vi "Volume_Naming.vi"() -> (5 "Plug in titles":string[](array[string]), 7 "Plug in values":string[](array[string]))   [LabVIEW 2013]
uses:
  File/Setup_Filetype.ctl
  Globals/Meas_global.vi
panel:
  out "Volume File Present?":bool=TRUE
  out "Values":string[](array[string])
  out "Output Position":dbl[](array[numeric])
  out "Zmin":dbl
  out "Ymin":dbl
  out "Zmax":dbl
  out "Ymax":dbl
  out "Z":dbl
  out "Volume Name":string
  out "Y":dbl
  out "X":dbl
  out "Row number":i32
  out "Xmin":dbl
  out "Xmax":dbl
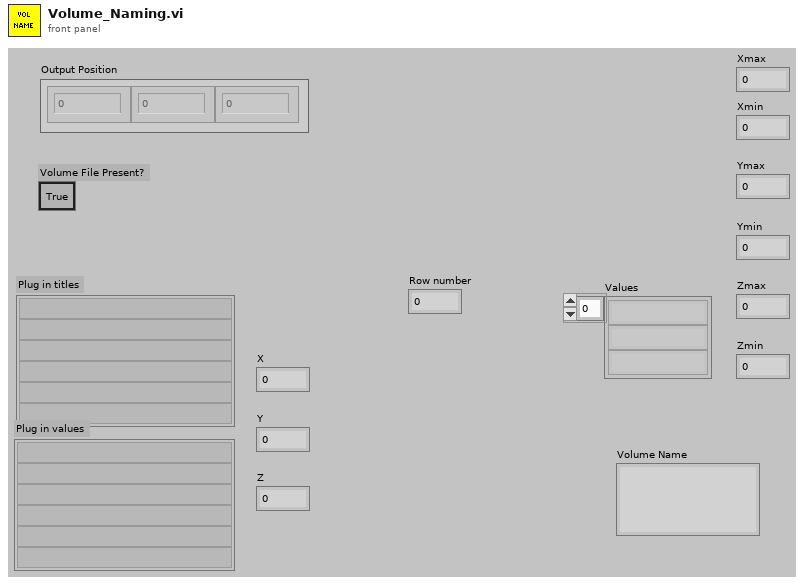
[diagram p1: front panel]
types:
  T1 = typedef "Setup_Filetype.ctl" = enum16{"Measurement Setups", "Calibration Setups", "General", "Results File Plotter Setups", "Speed Calib Tweaks"}
  T2 = enum16{"To Traverse Coordinates", "To User Coordinates"}
  T3 = typedef "Post_Process.ctl" = enum16{"Take New Data", "Post Process Raw Data File"}
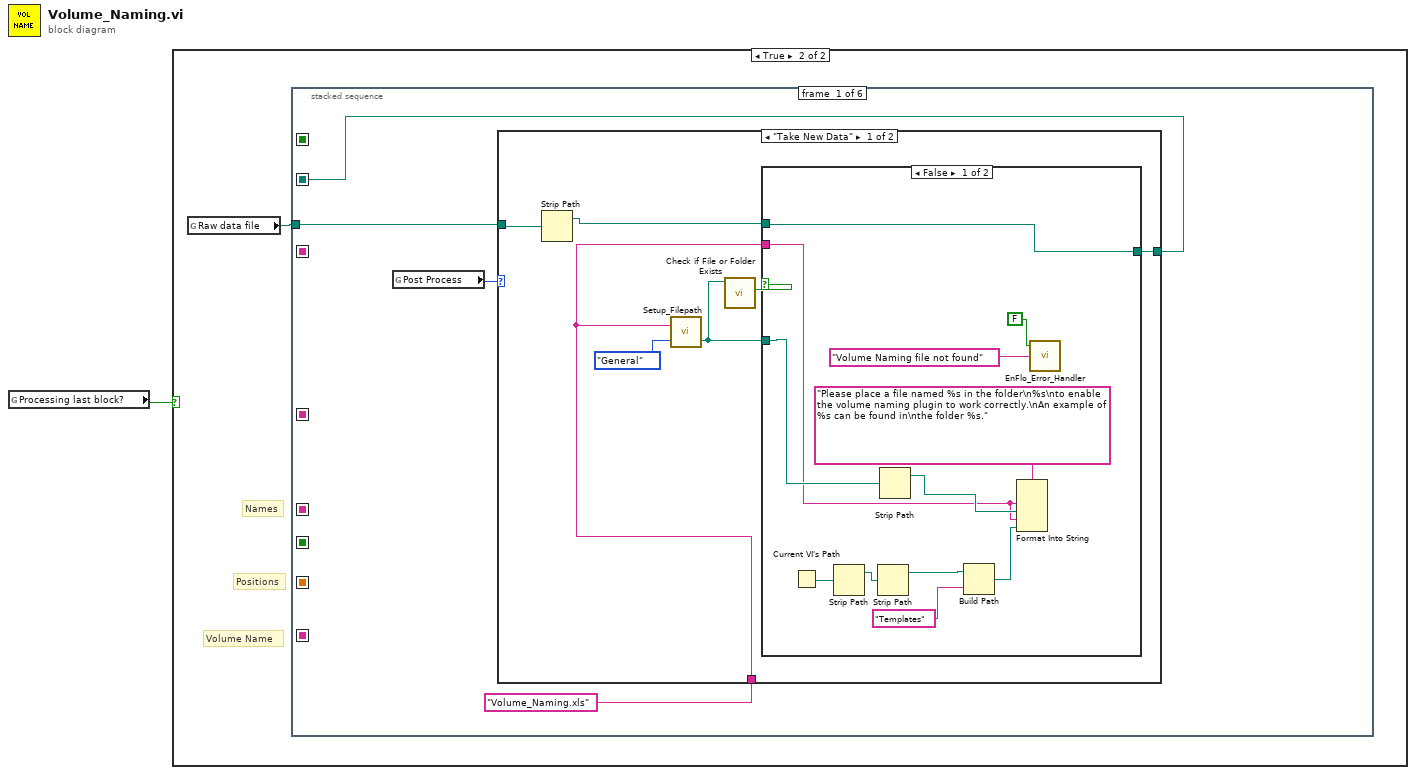
[diagram p0: block diagram]
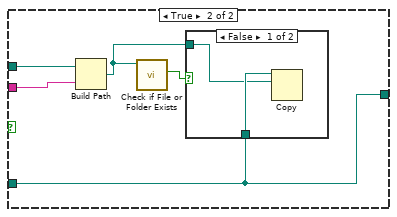
[diagram p3: hidden frame]
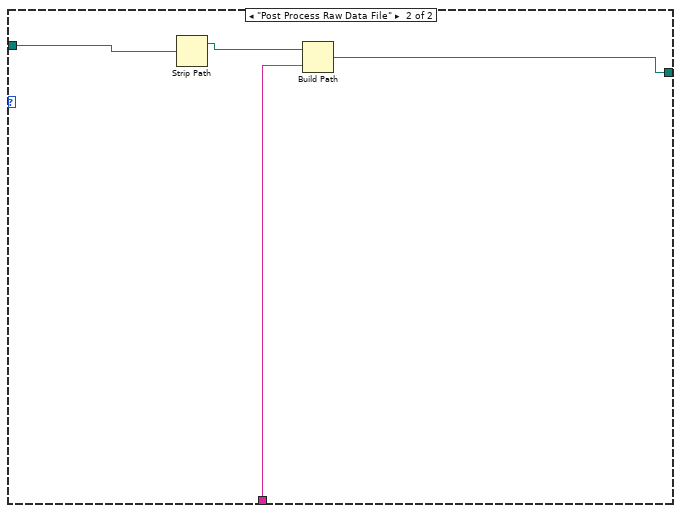
[diagram p5: hidden frame]
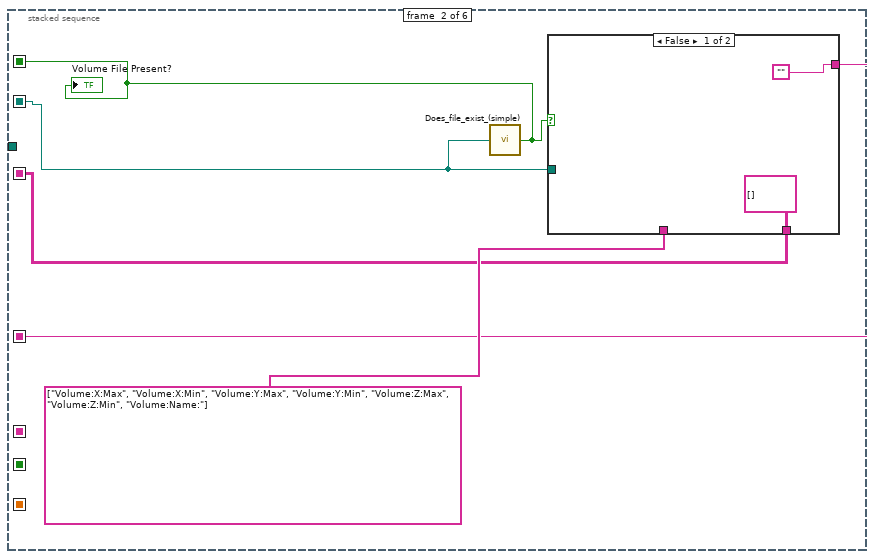
[diagram p6: hidden frame]
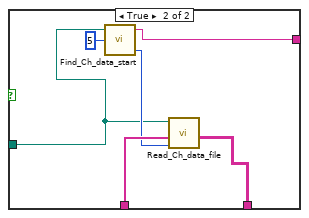
[diagram p7: hidden frame]
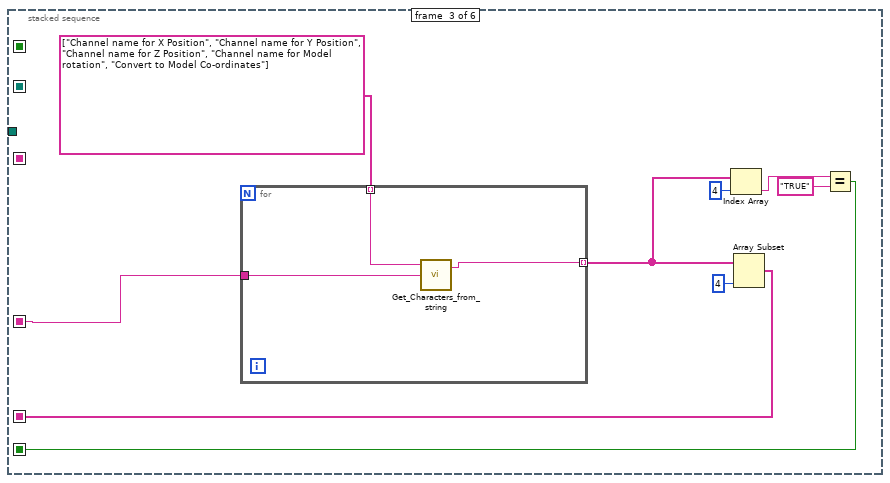
[diagram p8: hidden frame]
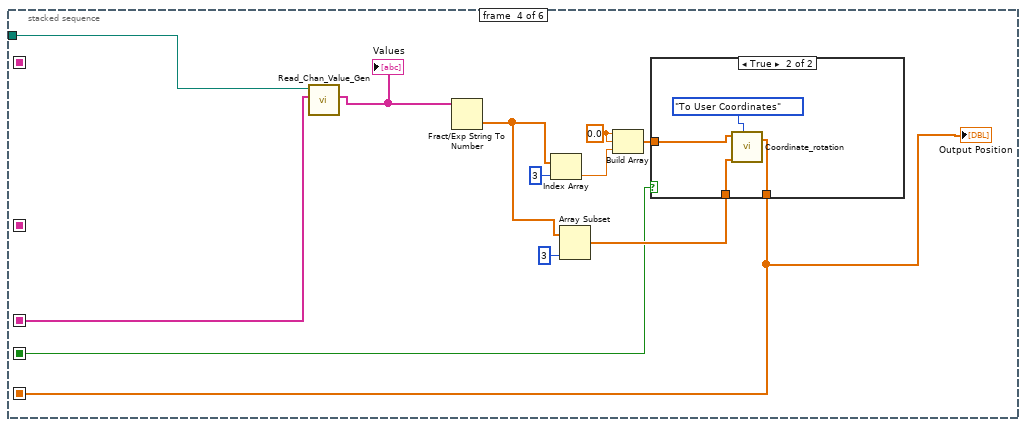
[diagram p9: hidden frame]
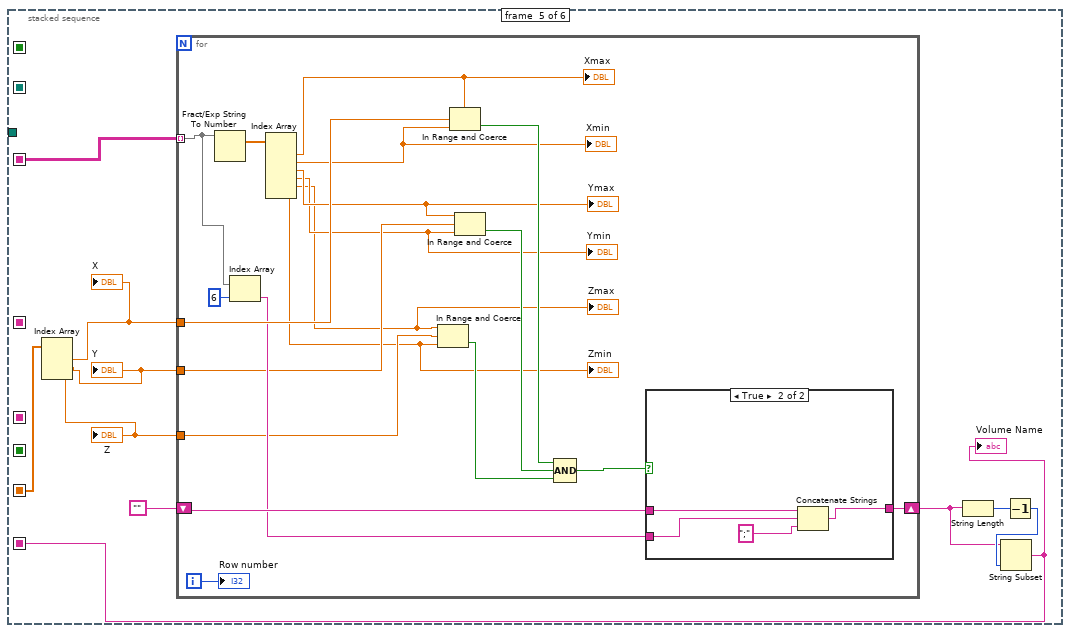
[diagram p11: hidden frame]
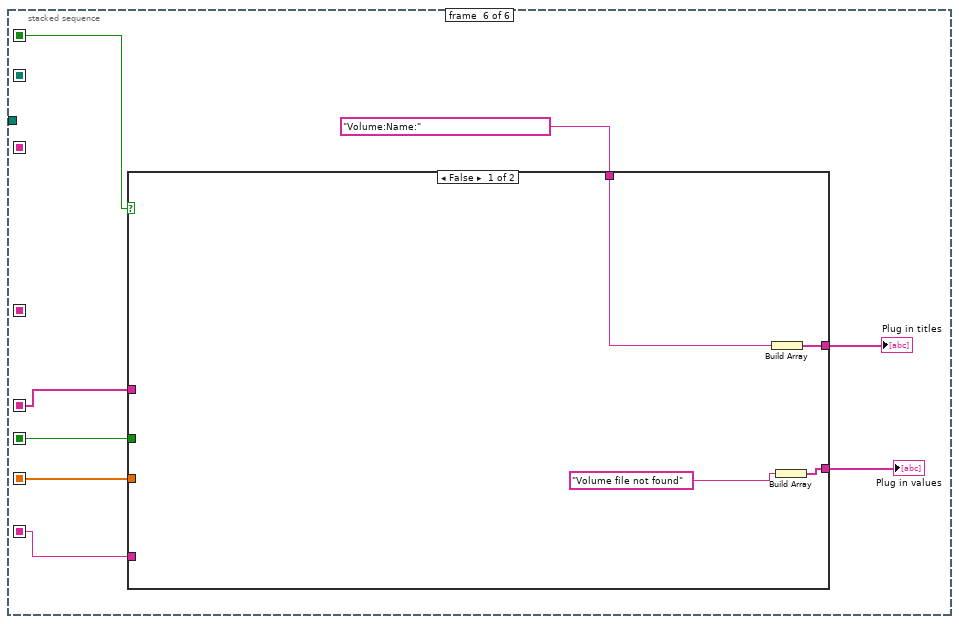
[diagram p13: hidden frame]
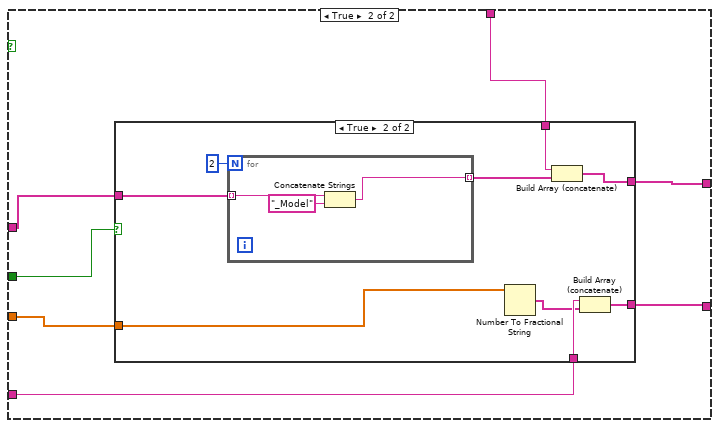
[diagram p14: hidden frame]
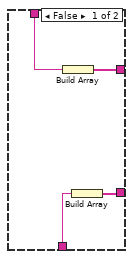
[diagram p15: hidden frame]
diagram:
  n1 = global read "Meas_global.vi" "Processing last block?"() -> (w1:bool)
  n2 = case shown="True" w1 {
    frame False {
    }
    frame True {
      # "Volume Name"
      # "Positions"
      # "Names"
      n3 = global read "Meas_global.vi" "Raw data file"() -> (w2:path)
      n4 = stacked-sequence {
        seq-local: [_ w40 _ _ _ _] -> [_ _ _ _ w88 _]
        seq-local: [_ _ _ w63 _ _] -> [_ _ _ _ w86 w121]
        seq-local: [_ _ _ _ w79 _] -> [_ _ _ _ _ w119]
        seq-local: [_ w39 _ _ _ _] -> [_ _ w58 _ _ _]
        seq-local: [_ _ w55 _ _ _] -> [_ _ _ w65 _ w116]
        seq-local: [_ _ w50 _ _ _] -> [_ _ _ w64 _ w120]
        seq-local: [_ w38 _ _ _ _] -> [_ _ _ _ _ w115]
        seq-local: [w5 _ _ _ _ _] -> [_ w37 _ _ _ _]
        tunnel: w2 -> [w4 _ _ w62 _ _]
        frame #0 {
          n5 = global read "Meas_global.vi" "Post Process"() -> (w6:T3)
          n6 = case shown="\"Take New Data\"" w6 {
            tunnel: [w7 w33] -> w5
            tunnel: w4 -> [w12 w35]
            tunnel: "Volume_Naming.xls" ("name or relative path") -> [w10 w34]
            frame "Take New Data" {
              n7 = Strip Path(path=w12) -> (stripped path=w11:path)  [unwired: 1 out]
              n8 = call "Setup_Filepath.vi"("Setup File Type"=Setup_Filetype."General", "Filename in"=w10) -> ("Filename Out"=w9:path)  [unwired: 1 out]
              n9 = call <vilib>:"Check if File or Folder Exists.vi"("path"=w9) -> ("file or folder exists?"=w8:bool)  [unwired: 8 in, 2 out]
              n10 = case shown="False" w8 {
                tunnel: w11 -> [w14 w30]
                tunnel: w10 -> [w20 w29]
                tunnel: w9 -> [w22 w26]
                tunnel: [w14 w26] -> w7
                frame False {
                  n11 = Current VI's Path() -> (path=w19:path)
                  n12 = Strip Path(path=w19) -> (stripped path=w18:path)  [unwired: 1 out]
                  n13 = Strip Path(path=w18) -> (stripped path=w17:path)  [unwired: 1 out]
                  n14 = Strip Path(path=w22) -> (stripped path=w21:path)  [unwired: 1 out]
                  n15 = Build Path(base path=w17, name or relative path="Templates") -> (appended path=w15:path)
                  n16 = Format Into String(format string="Please place a file named %s in the folder\n%s\nto enable the volume naming plugin to work correctly.\nAn example of %s can be found in\nthe folder %s.", w20, w21, w20, w15) -> ()  [unwired: 2 in, 2 out]
                  n17 = call "EnFlo_Error_Handler.vi"("Error Type"="Volume Naming file not found", "Dialog Box (T)"=FALSE) -> ()  [unwired: 1 in, 3 out]
                }
                frame True {
                  n18 = Build Path(base path=w30, name or relative path=w29) -> (appended path=w27:path)
                  n19 = call <vilib>:"Check if File or Folder Exists.vi"("path"=w27) -> ("file or folder exists?"=w28:bool)  [unwired: 8 in, 2 out]
                  n20 = case shown="False" w28 {
                    tunnel: w26 -> [w32 _]
                    tunnel: w27 -> [w31 _]
                    frame False {
                      n21 = Copy(10:w31, 11:w32) -> ()  [unwired: 3 in, 3 out]
                    }
                    frame True {
                    }
                  }
                }
              }
            }
            frame "Post Process Raw Data File" {
              n22 = Strip Path(path=w35) -> (stripped path=w36:path)  [unwired: 1 out]
              n23 = Build Path(base path=w36, name or relative path=w34) -> (appended path=w33:path)
            }
          }
        }
        frame #1 {
          n24 = call "Does_file_exist_(simple).vi"("Pathname"=w37) -> ("exists?"=w38:bool)
          "Volume File Present?" <- w38
          n25 = case shown="False" w38 {
            tunnel: string[] ["Volume:X:Max", "Volume:X:Min", "Volume:Y:Max", "Volume:Y:Min", "Volume:Z:Max", "Volume:Z:Min", "Volume:Name:"] ("Ch names Out") -> [_ w49]
            tunnel: [string[][] [] ("Channel Values") w48] -> w40
            tunnel: ["" w47] -> w39
            tunnel: w37 -> [_ w44]
            frame False {
            }
            frame True {
              n26 = call "Find_Ch_data_start.vi"("Approx No Of Columns"=5, "Filename"=w44) -> ("Start of read offset output"=w45:i32, "String before data"=w47:string)  [unwired: 1 in, 1 out]
              n27 = call "Read_Ch_data_file.vi"("Start of read offset (chars.: 0)"=w45, "Present Channels"=w49, "Filename"=w44) -> ("Channel Values"=w48:string[][])  [unwired: 2 in, 4 out]
            }
          }
        }
        frame #2 {
          n28 = for {
            tunnel: w58 -> [w61]
            tunnel: string[] ["Channel name for X Position", "Channel name for Y Position", "Channel name for Z Position", "Channel name for Model rotation", "Convert to Model Co-ordinates"] -> [w60] mode=indexing
            tunnel: [w59] -> w54 mode=indexing
            n29 = call "Get_Characters_from_string.vi"("Input string"=w61, "Variable name"=w60) -> ("Value"=w59:string)  [unwired: 1 in, 1 out]
          }
          n30 = Index Array(array=w54, index=4) -> (element=w52:string)
          n31 = Array Subset(array=w54, length=4) -> (w55:string[])  [unwired: 1 in]
          n32 = Equal?(x=w52, y="TRUE") -> (x = y?=w50:bool)
        }
        frame #3 {
          w70 = 0.0 ("element")
          n33 = call "Read_Chan_Value_Gen.vi"("Desired Ch Names"=w65, "Raw data file"=w62) -> ("Values"=w73:string[])  [unwired: 9 in]
          "Values" <- w73
          n34 = Fract/Exp String To Number(string=w73) -> (number=w68:dbl[])  [unwired: 3 in, 1 out]
          n35 = Index Array(array=w68, index=3) -> (element=w71:dbl)
          n36 = Array Subset(array=w68, length=3) -> (w66:dbl[])  [unwired: 1 in]
          n37 = Build Array(w70, w70, w71) -> (w69:dbl[])
          n38 = case shown="True" w64 {
            tunnel: w69 -> [_ w77]
            tunnel: w66 -> [w74 w76]
            tunnel: [w74 w75] -> w63
            frame False {
            }
            frame True {
              n39 = call "Coordinate_rotation.vi"("Model       Roll      Pitch       Yaw (deg)"=w77, "Input Position"=w76, "Mode"=T2."To User Coordinates") -> ("Output Position"=w75:dbl[])  [unwired: 2 in, 1 out]
            }
          }
          "Output Position" <- w63
        }
        frame #4 {
          n40 = Index Array(array=w86) -> (element #1=w85:dbl, element #2=w84:dbl, element #3=w83:dbl)  [unwired: 3 in]
          "X" <- w85
          "Y" <- w84
          "Z" <- w83
          n41 = for {
            tunnel: w88 -> [w106] mode=indexing
            tunnel: w85 -> [w103]
            shift-right: [w98] -> w80
            shift-left: "" -> [w100]
            tunnel: w84 -> [w94]
            tunnel: w83 -> [w92]
            i -> [w108]
            n42 = Fract/Exp String To Number(string=w106) -> (number=w107:dbl[])  [unwired: 3 in, 1 out]
            n43 = Index Array(array=w106, index=6) -> (element=w99:string)
            n44 = Index Array(array=w107) -> (element #1=w104:dbl, element #2=w97:dbl, element #3=w95:dbl, element #4=w93:dbl, element #5=w89:dbl, element #6=w90:dbl)  [unwired: 6 in]
            "Xmax" <- w104
            "Xmin" <- w97
            "Ymax" <- w95
            "Zmax" <- w89
            "Ymin" <- w93
            "Zmin" <- w90
            n45 = In Range and Coerce(upper limit=w89, x=w92, lower limit=w90) -> (In Range?=w91:bool)  [unwired: 1 out]
            n46 = In Range and Coerce(upper limit=w104, x=w103, lower limit=w97) -> (In Range?=w102:bool)  [unwired: 1 out]
            n47 = In Range and Coerce(upper limit=w95, x=w94, lower limit=w93) -> (In Range?=w96:bool)  [unwired: 1 out]
            n48 = Compound Arithmetic op=AND(w102, w96, w91) -> (w101:bool)
            n49 = case shown="True" w101 {
              tunnel: w100 -> [w109 w113]
              tunnel: w99 -> [_ w112]
              tunnel: [w109 w110] -> w98
              frame False {
              }
              frame True {
                n50 = Concatenate Strings(w113, w112, ";") -> (w110:string)
              }
            }
            "Row number" <- w108
          }
          n51 = String Length(string=w80) -> (length=w82:i32)
          n52 = Decrement(x=w82) -> (x-1=w81:i32)
          n53 = String Subset(string=w80, length (rest)=w81) -> (substring=w79:string)  [unwired: 1 in]
          "Volume Name" <- w79
        }
        frame #5 {
          n54 = case shown="False" w115 {
            tunnel: w121 -> [_ w132]
            tunnel: w120 -> [_ w131]
            tunnel: w119 -> [_ w130]
            tunnel: [w124 w129] -> w118
            tunnel: [w123 w128] -> w117
            tunnel: w116 -> [_ w127]
            tunnel: "Volume:Name:" -> [w125 w126]
            frame False {
              n55 = Build Array(w125) -> (w124:string[])
              n56 = Build Array("Volume file not found") -> (w123:string[])
            }
            frame True {
              n57 = case shown="True" w131 {
                tunnel: w132 -> [_ w145]
                tunnel: w126 -> [w136 w144]
                tunnel: w130 -> [w133 w143]
                tunnel: [w135 w141] -> w129
                tunnel: [w134 w140] -> w128
                tunnel: w127 -> [_ w138]
                frame False {
                  n58 = Build Array(w136) -> (w135:string[])
                  n59 = Build Array(w133) -> (w134:string[])
                }
                frame True {
                  n60 = for {
                    N: 2 -> [_]
                    tunnel: w138 -> [w148] mode=indexing
                    tunnel: [w146] -> w137 mode=indexing
                    n61 = Concatenate Strings(w148, "_Model" ("string")) -> (w146:string)
                  }
                  n62 = Number To Fractional String(number=w145) -> (F-format string=w142:string[])  [unwired: 3 in]
                  n63 = Build Array (concatenate)(w144, w137) -> (w141:string[])
                  n64 = Build Array (concatenate)(w143, w142) -> (w140:string[])
                }
              }
            }
          }
          "Plug in values" <- w117
          "Plug in titles" <- w118
        }
      }
    }
  }
